vi "LM3Sxxxx_ADC_Specify_Node.vi"(10 "Node Attributes":T2) -> (3 "type out":T1)   [LabVIEW 2011]
uses:
  <vilib>/Embedded/ARM/LM3Sxxxx/ADC/LM3Sxxxx_ADC_Node_Attr.ctl
  <vilib>/eio/EIO_TypeDescriptor.ctl
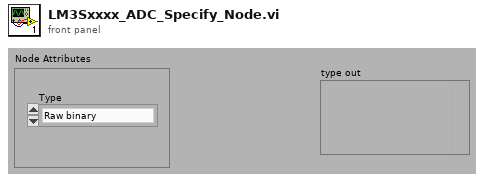
[diagram p1: front panel]
types:
  T1 = typedef "EIO_TypeDescriptor.ctl" = variant
  T2 = typedef "LM3Sxxxx_ADC_Node_Attr.ctl" = cluster{"Type":enum16{"Raw binary", "Scaled Volts"}}
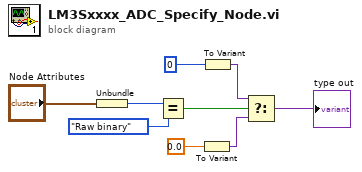
[diagram p0: block diagram]
diagram:
  n1 = Unbundle("Node Attributes") -> ("Type"=w8:enum16{"Raw binary", "Scaled Volts"})
  n2 = Equal?(x=w8, y=enum16{"Raw binary", "Scaled Volts"}."Raw binary") -> (x = y?=w2:bool)
  n3 = To Variant(anything=0.0) -> (Variant=w4:variant)
  n4 = To Variant(anything=u32 0) -> (Variant=w6:variant)
  n5 = Select(t=w6, s=w2, f=w4) -> (s? t:f=→"type out":variant)
